vi "Get SN and Cal Date.vi"(8 "error in (no error)":errorcluster, 11 "ENET_BS1200 in":refnum<class "ENET_BS1200.lvclass">) -> (0 "error out":errorcluster, 1 "Calibration Date":timestamp, 2 "Serial Number":string, 3 "ENET_BS1200 out":refnum<class "ENET_BS1200.lvclass">)   [LabVIEW 2021, in "BS120x Driver.lvlib" / "ENET_BS1200.lvclass"]
uses:
  ENET_BS1200.lvclass
  TypeDefs/Protocol.ctl
  <vilib>/WebDAVClient/Advanced/Get Buffer.vi
  BS120x.lvclass
  <vilib>/WebDAVClient/NI_WebDAV.lvlib
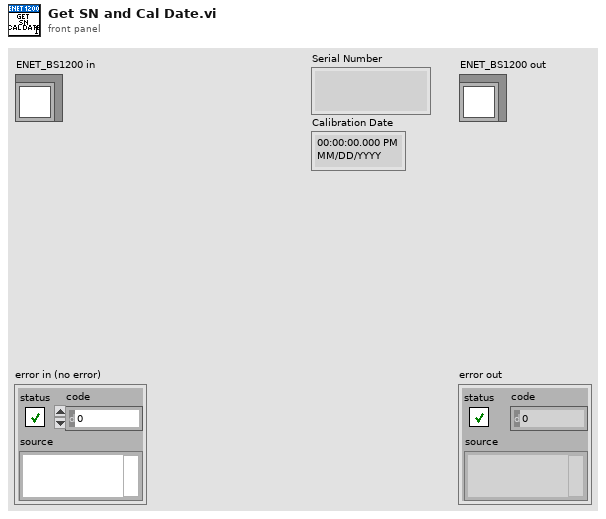
[diagram p1: front panel]
types:
  T1 = typedef "NI_WebDAV.lvlib/SessionHandle.ctl" = refnum<k1>
  T2 = typedef "BS120x Driver.lvlib/BS120x.lvclass/Protocol.ctl" = enum16{"CAN", "Ethernet"}
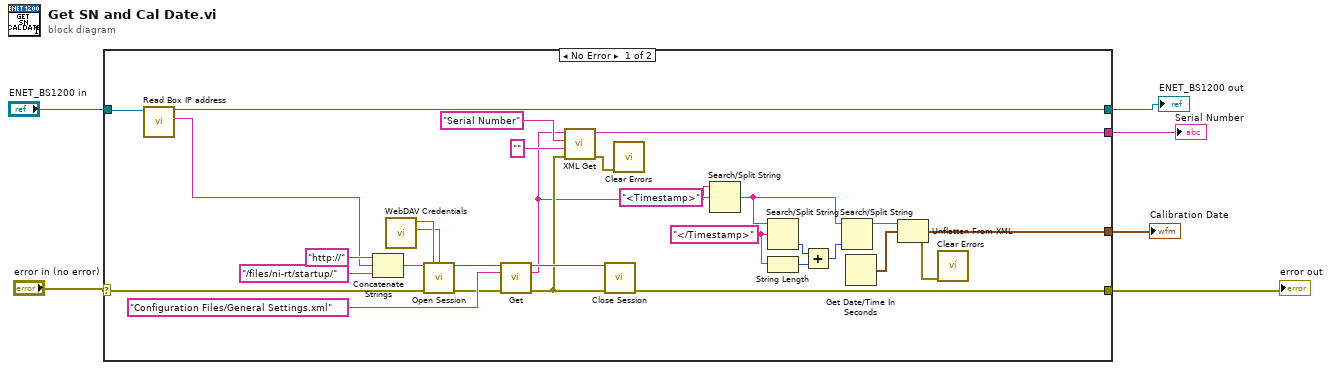
[diagram p0: block diagram]
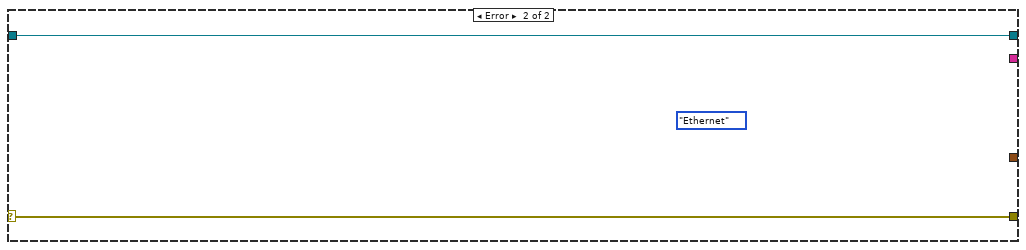
[diagram p2: hidden frame]
diagram:
  n1 = case shown="No Error" "error in (no error)" {
    selector: "error in (no error)" -> [w34 w38]
    tunnel: [w27 w38] -> w2
    tunnel: [w22 w37] -> w1
    tunnel: "ENET_BS1200 in" -> [w23 w37]
    tunnel: [w20 _] -> w4
    tunnel: [w8 _] -> w3
    frame No Error {
      w17 = "</Timestamp>" ("search string/char (-)")
      n2 = call-dynamic "Read Box IP address.vi"("ENET_BS120x in"=w23) -> ("Box IP address"=w21:string, "ENET_BS120x out"=w22:refnum<class "ENET_BS1200.lvclass">)  [unwired: 8 in, 1 out]
      n3 = Concatenate Strings("http://" ("string"), w21, "/files/ni-rt/startup/" ("string")) -> (w31:string)
      n4 = call "WebDAV Credentials.vi"() -> ("Password"=w32:string, "Username"=w33:string)  [unwired: 10 in]
      n5 = call <vilib>:"Open Session.vi"("host uri prefix"=w31, "username"=w33, "password"=w32, "error in (no error)"=w34) -> ("session handle out"=w26:T1, "error out"=w25:errorcluster)  [unwired: 10 in]
      n6 = call-poly <vilib>:"Get.vi"("session handle"=w26, "relative uri"="Configuration Files/General Settings.xml" ("string"), "error in (no error)"=w25) -> ("session handle out"=w24:T1, "data"=w9:string, "error out"=w19:errorcluster)  [unwired: 10 in]
      n7 = call "XML Get.vi"("error in (no error)"=w19, "Data Type"="" ("regular expression"), "Parameter"="Serial Number" ("regular expression"), "XML String in"=w9) -> ("error out"=w7:errorcluster, "Value"=w20:string)  [unwired: 6 in]
      n8 = call <vilib>:"Close Session.vi"("session handle"=w24, "error in (no error)"=w19) -> ("error out"=w27:errorcluster)  [unwired: 13 in]
      n9 = call <vilib>:"Clear Errors.vi"("error in (no error)"=w7) -> ()  [unwired: 5 in, 2 out]
      n10 = Search/Split String(string=w9, search string/char (-)="<Timestamp>" ("regular expression")) -> (match + rest of string=w14:string)  [unwired: 1 in, 2 out]
      n11 = Search/Split String(string=w14, search string/char (-)=w17) -> (offset of match=w15:i32)  [unwired: 1 in, 2 out]
      n12 = String Length(string=w17) -> (length=w16:i32)
      n13 = Add(x=w15, y=w16) -> (x+y=w13:i32)
      n14 = Search/Split String(string=w14, offset (0)=w13) -> (substring before match=w12:string)  [unwired: 1 in, 2 out]
      n15 = Get Date/Time In Seconds() -> (seconds since 1Jan1904=w11:timestamp)
      n16 = Unflatten From XML(xml string=w12, type=w11) -> (value=w8:timestamp, error out=w10:errorcluster)  [unwired: 1 in]
      n17 = call <vilib>:"Clear Errors.vi"("error in (no error)"=w10) -> ()  [unwired: 5 in, 2 out]
    }
    frame Error {
      (unwired) Protocol."Ethernet" ("Protocol")
    }
  }
  "error out" <- w2
  "ENET_BS1200 out" <- w1
  "Serial Number" <- w4
  "Calibration Date" <- w3
